vi "hex display to normal display.vi"(10 "Hex display":string) -> (1 "Normal display":string)   [LabVIEW 2015]
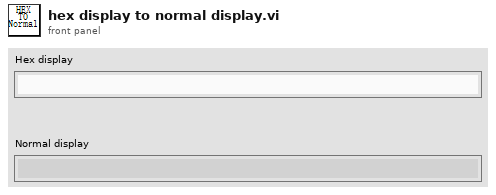
[diagram p1: front panel]
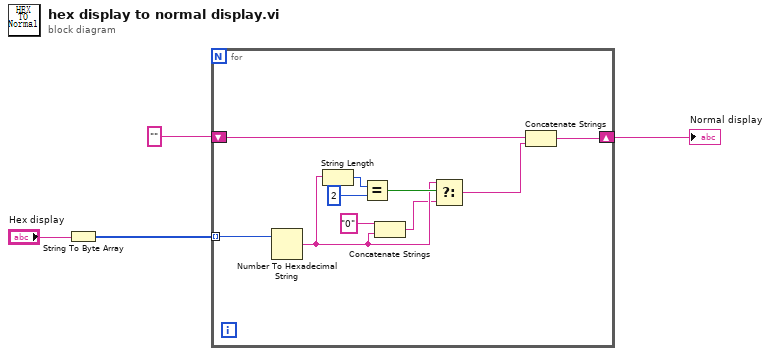
[diagram p0: block diagram]
diagram:
  n1 = String To Byte Array(string="Hex display") -> (unsigned byte array=w3:u8[])
  n2 = for {
    tunnel: w3 -> [w14] mode=indexing
    shift-right: [w7] -> w1
    shift-left: "" -> [w5]
    n3 = Number To Hexadecimal String(2:w14) -> (0:w9:string)  [unwired: 1 in]
    n4 = String Length(string=w9) -> (length=w13:i32)
    n5 = Equal?(x=w13, y=2) -> (x = y?=w11:bool)
    n6 = Concatenate Strings("0", w9) -> (w8:string)
    n7 = Select(t=w9, s=w11, f=w8) -> (s? t:f=w6:string)
    n8 = Concatenate Strings(w5, w6) -> (w7:string)
  }
  "Normal display" <- w1
